vi "GUI.Button.btn_FindDevices.vi"(8 "error in (no error)":errorcluster, 10 "isSearching? (false)":bool) -> (0 "error out":errorcluster)   [LabVIEW 2019]
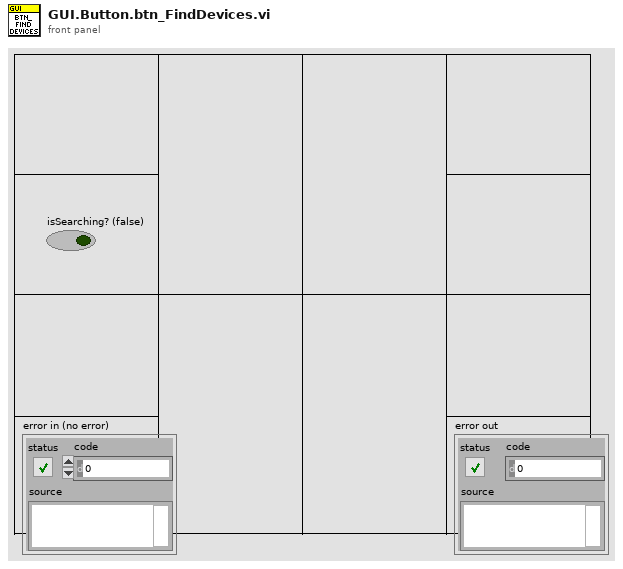
[diagram p1: front panel]
types:
  T1 = enum8{"Enabled", "Disabled", "Disabled and Grayed Out"}
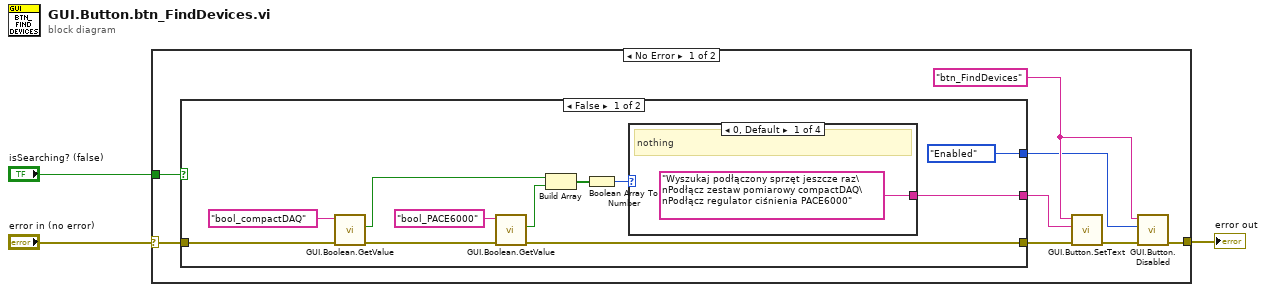
[diagram p0: block diagram]
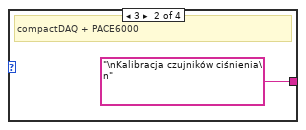
[diagram p2: hidden frame]
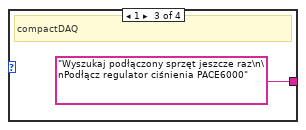
[diagram p3: hidden frame]
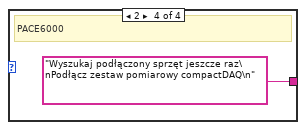
[diagram p4: hidden frame]
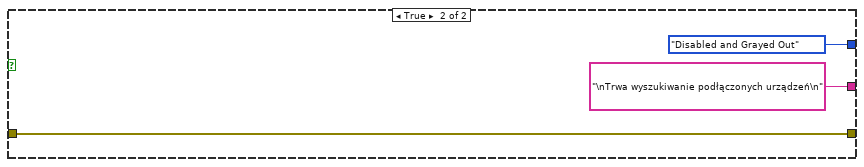
[diagram p5: hidden frame]
diagram:
  n1 = case shown="No Error" "error in (no error)" {
    selector: "error in (no error)" -> [w5 w30]
    tunnel: [w10 w30] -> w1
    tunnel: "isSearching? (false)" -> [w8 _]
    frame No Error {
      w7 = "btn_FindDevices"
      n2 = case shown="False" w8 {
        tunnel: [w15 "\nTrwa wyszukiwanie podłączonych urządzeń\n"] -> w9
        tunnel: [T1."Enabled" ("buttonDisabled") T1."Disabled and Grayed Out" ("buttonDisabled")] -> w6
        tunnel: w5 -> [w19 w27]
        tunnel: [w14 w27] -> w4
        frame False {
          n3 = call "GUI.Boolean.GetValue.vi"("error in (no error)"=w19, "booleanName"="bool_compactDAQ") -> ("error out"=w21:errorcluster, "booleanValue"=w17:bool)  [unwired: 8 in]
          n4 = call "GUI.Boolean.GetValue.vi"("error in (no error)"=w21, "booleanName"="bool_PACE6000") -> ("error out"=w14:errorcluster, "booleanValue"=w16:bool)  [unwired: 8 in]
          n5 = Build Array(w17, w16) -> (w18:bool[])
          n6 = Boolean Array To Number(Boolean array=w18) -> (number=w13:u32)
          n7 = case shown="0, Default" w13 {
            tunnel: ["Wyszukaj podłączony sprzęt jeszcze raz\nPodłącz zestaw pomiarowy compactDAQ\nPodłącz regulator ciśnienia PACE6000" ("controlBoolText") "\nKalibracja czujników ciśnienia\n" ("controlBoolText") "Wyszukaj podłączony sprzęt jeszcze raz\n\nPodłącz regulator ciśnienia PACE6000" ("controlBoolText") "Wyszukaj podłączony sprzęt jeszcze raz\nPodłącz zestaw pomiarowy compactDAQ\n" ("controlBoolText")] -> w15
            frame 0, Default {
              # "nothing"
            }
            frame 3 {
              # "compactDAQ + PACE6000"
            }
            frame 1 {
              # "compactDAQ"
            }
            frame 2 {
              # "PACE6000"
            }
          }
        }
        frame True {
        }
      }
      n8 = call "GUI.Button.SetText.vi"("error in (no error)"=w4, "buttonText"=w9, "buttonName"=w7) -> ("error out"=w11:errorcluster)  [unwired: 8 in]
      n9 = call "GUI.Button.Disabled.vi"("error in (no error)"=w11, "buttonDisabled"=w6, "buttonName"=w7) -> ("error out"=w10:errorcluster)  [unwired: 8 in]
    }
    frame Error {
    }
  }
  "error out" <- w1
